vi "getNotifierServerStatus_tel.vi"(8 "error in (no error)":errorcluster, 10 "Timeout Notifier":i32, 11 "TcpServerTel in":refnum<class "TcpServerTel.lvclass">) -> (0 "error out":errorcluster, 1 "connStatus":bool, 2 "connStatusCluster":T1, 3 "TcpServerTel out":refnum<class "TcpServerTel.lvclass">)   [LabVIEW 2018, in "TcpServerTel.lvclass"]
doc: "Get the notifierServerStatus from TcpServerTel.tcpServerStateMachine.vi. The notifier will inform the user if the command server disconnects or reconnects to the client. This vi is needed to avoid to expose the TcpServerBase.getNotifierServerStatus.vi to the user."
uses:
  TcpServerTel.lvclass
  home/pcortes/Documents/github/ts_labview_tcp_json/src/TcpServerBase/TcpServerBase.lvclass
  TcpServerBase/TcpServerBase.lvclass
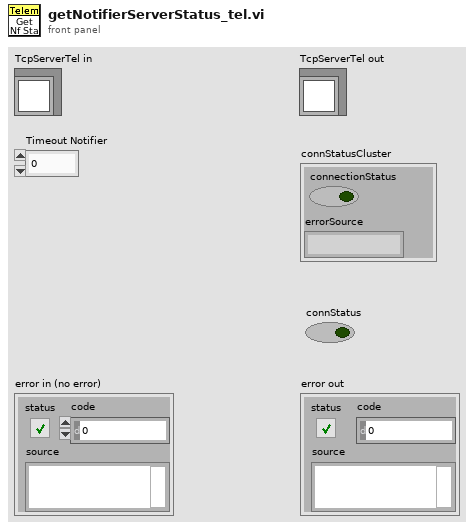
[diagram p1: front panel]
types:
  T1 = cluster{"connectionStatus":bool, "errorSource":string}
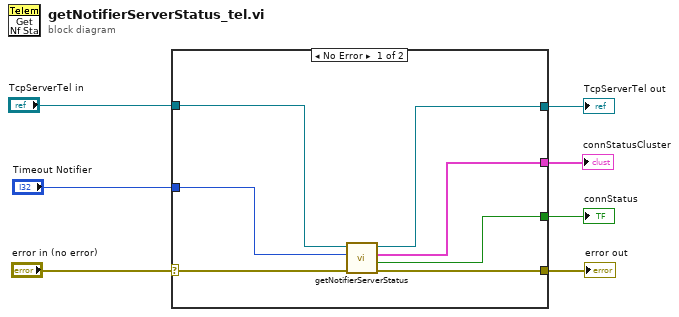
[diagram p0: block diagram]
diagram:
  n1 = case shown="No Error" "error in (no error)" {
    selector: "error in (no error)" -> [w14 w16]
    tunnel: "Timeout Notifier" -> [w10 _]
    tunnel: "TcpServerTel in" -> [w12 w15]
    tunnel: [w13 w16] -> w4
    tunnel: [w9 _] -> w3
    tunnel: [w8 _] -> w2
    tunnel: [w11 w15] -> w1
    frame No Error {
      n2 = call "getNotifierServerStatus.vi"("error in (no error)"=w14, "notifier timeout"=w10, "TcpServerBase in"=w12) -> ("error out"=w13:errorcluster, "timeout?"=w8:bool, "connStatusCluster"=w9:T1, "TcpServerBase out"=w11:refnum<class "TcpServerTel.lvclass">)  [unwired: 5 in]
    }
    frame Error {
    }
  }
  "error out" <- w4
  "connStatusCluster" <- w3
  "connStatus" <- w2
  "TcpServerTel out" <- w1
